vi "超标留样流程.vi"   [LabVIEW 2016]
types:
  T1 = enum16{"德润DR803M", "德润DR803L", "德润DR803F", "科盛超标留样"}
  T2 = enum32{"Bad", "Idle", "Run top level", "Running"}
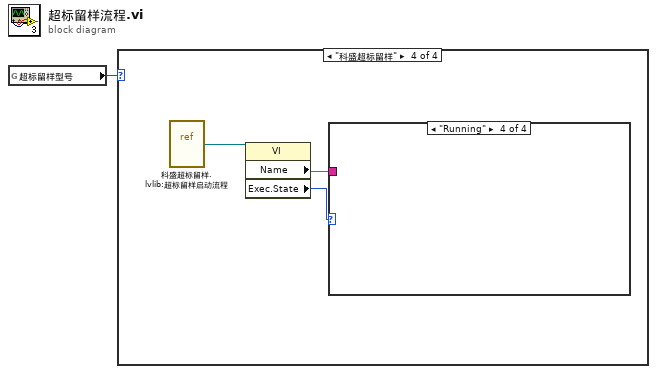
[diagram p0: block diagram]
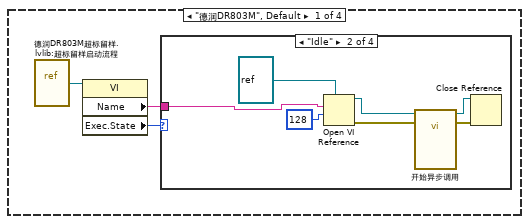
[diagram p2: hidden frame]
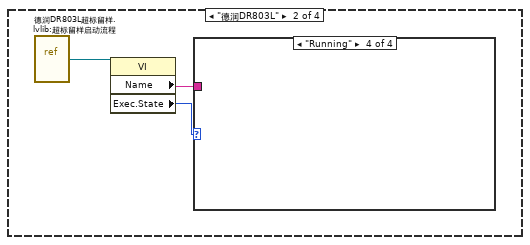
[diagram p6: hidden frame]
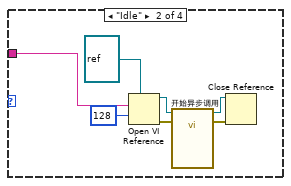
[diagram p8: hidden frame]
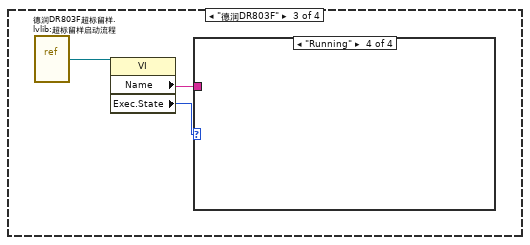
[diagram p10: hidden frame]
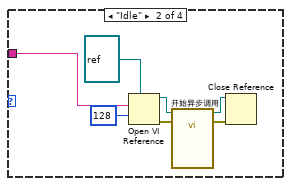
[diagram p12: hidden frame]
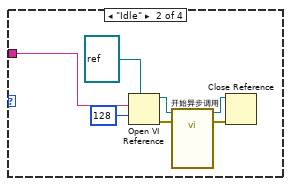
[diagram p15: hidden frame]
diagram:
  n1 = global read "断电保存全局.vi" "超标留样型号"() -> (w1:T1)
  n2 = case shown="\"科盛超标留样\"" w1 {
    frame "德润DR803M", Default {
      n3 = vi-ref "德润DR803M超标留样.lvlib:超标留样启动流程.vi"() -> (w2:refnum<vi>)
      n4 = property class="VI"(reference=w2) -> ("Name"=w3:string, "Exec.State"=w4:T2)  [unwired: 1 in, 2 out]
      n5 = case shown="\"Idle\"" w4 {
        tunnel: w3 -> [_ w7 _ _]
        frame "Bad", Default {
        }
        frame "Idle" {
          n6 = Open VI Reference(type specifier VI Refnum (for type only)=refnum<vi> refnum ("类型说明符VI引用句柄（仅用于类型）"), vi path=w7, options=128 ("选项")) -> (vi reference=w11:refnum<vi>, error out=w6:errorcluster)  [unwired: 3 in]
          n7 = call-by-ref "开始异步调用"(reference=w11, error in=w6) -> (reference out=w10:refnum<vi>, error out=w5:errorcluster)  [unwired: 12 in]
          n8 = Close Reference(reference=w10, error in (no error)=w5) -> ()  [unwired: 1 out]
        }
        frame "Run top level" {
        }
        frame "Running" {
        }
      }
    }
    frame "德润DR803L" {
      n9 = vi-ref "德润DR803L超标留样.lvlib:超标留样启动流程.vi"() -> (w14:refnum<vi>)
      n10 = property class="VI"(reference=w14) -> ("Name"=w13:string, "Exec.State"=w12:T2)  [unwired: 1 in, 2 out]
      n11 = case shown="\"Running\"" w12 {
        tunnel: w13 -> [_ w17 _ _]
        frame "Bad", Default {
        }
        frame "Idle" {
          n12 = Open VI Reference(type specifier VI Refnum (for type only)=refnum<vi> refnum ("类型说明符VI引用句柄（仅用于类型）"), vi path=w17, options=128 ("选项")) -> (vi reference=w21:refnum<vi>, error out=w16:errorcluster)  [unwired: 3 in]
          n13 = call-by-ref "开始异步调用"(reference=w21, error in=w16) -> (reference out=w20:refnum<vi>, error out=w15:errorcluster)  [unwired: 12 in]
          n14 = Close Reference(reference=w20, error in (no error)=w15) -> ()  [unwired: 1 out]
        }
        frame "Run top level" {
        }
        frame "Running" {
        }
      }
    }
    frame "德润DR803F" {
      n15 = vi-ref "德润DR803F超标留样.lvlib:超标留样启动流程.vi"() -> (w22:refnum<vi>)
      n16 = property class="VI"(reference=w22) -> ("Name"=w23:string, "Exec.State"=w24:T2)  [unwired: 1 in, 2 out]
      n17 = case shown="\"Running\"" w24 {
        tunnel: w23 -> [_ w27 _ _]
        frame "Bad", Default {
        }
        frame "Idle" {
          n18 = Open VI Reference(type specifier VI Refnum (for type only)=refnum<vi> refnum ("类型说明符VI引用句柄（仅用于类型）"), vi path=w27, options=128 ("选项")) -> (vi reference=w31:refnum<vi>, error out=w26:errorcluster)  [unwired: 3 in]
          n19 = call-by-ref "开始异步调用"(reference=w31, error in=w26) -> (reference out=w30:refnum<vi>, error out=w25:errorcluster)  [unwired: 12 in]
          n20 = Close Reference(reference=w30, error in (no error)=w25) -> ()  [unwired: 1 out]
        }
        frame "Run top level" {
        }
        frame "Running" {
        }
      }
    }
    frame "科盛超标留样" {
      n21 = vi-ref "科盛超标留样.lvlib:超标留样启动流程.vi"() -> (w32:refnum<vi>)
      n22 = property class="VI"(reference=w32) -> ("Name"=w33:string, "Exec.State"=w34:T2)  [unwired: 1 in, 2 out]
      n23 = case shown="\"Running\"" w34 {
        tunnel: w33 -> [_ w37 _ _]
        frame "Bad", Default {
        }
        frame "Idle" {
          n24 = Open VI Reference(type specifier VI Refnum (for type only)=refnum<vi> refnum ("类型说明符VI引用句柄（仅用于类型）"), vi path=w37, options=128 ("选项")) -> (vi reference=w41:refnum<vi>, error out=w36:errorcluster)  [unwired: 3 in]
          n25 = call-by-ref "开始异步调用"(reference=w41, error in=w36) -> (reference out=w40:refnum<vi>, error out=w35:errorcluster)  [unwired: 12 in]
          n26 = Close Reference(reference=w40, error in (no error)=w35) -> ()  [unwired: 1 out]
        }
        frame "Run top level" {
        }
        frame "Running" {
        }
      }
    }
  }
